vi "GCSTranslateError.vi"(5 "error in":errorcluster) -> (14 "GCS Error?":bool, 15 "Error Description":string, 19 "error out":errorcluster)   [LabVIEW 2009]
doc: "Returns if error in contains a GCS error code and if this is the \ncase, it displays the corresponding error message and \nappends it to \"source\" in \"error out\".\n\nValid for all systems"
panel:
  # "Returns if error in contains a GCS error code and if this is the \ncase, it displays the corresponding error message and \nappends it to \"source\" in \"error out\"."
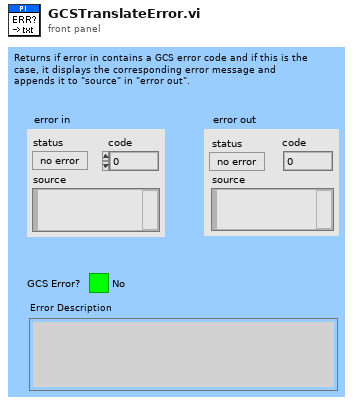
[diagram p1: front panel]
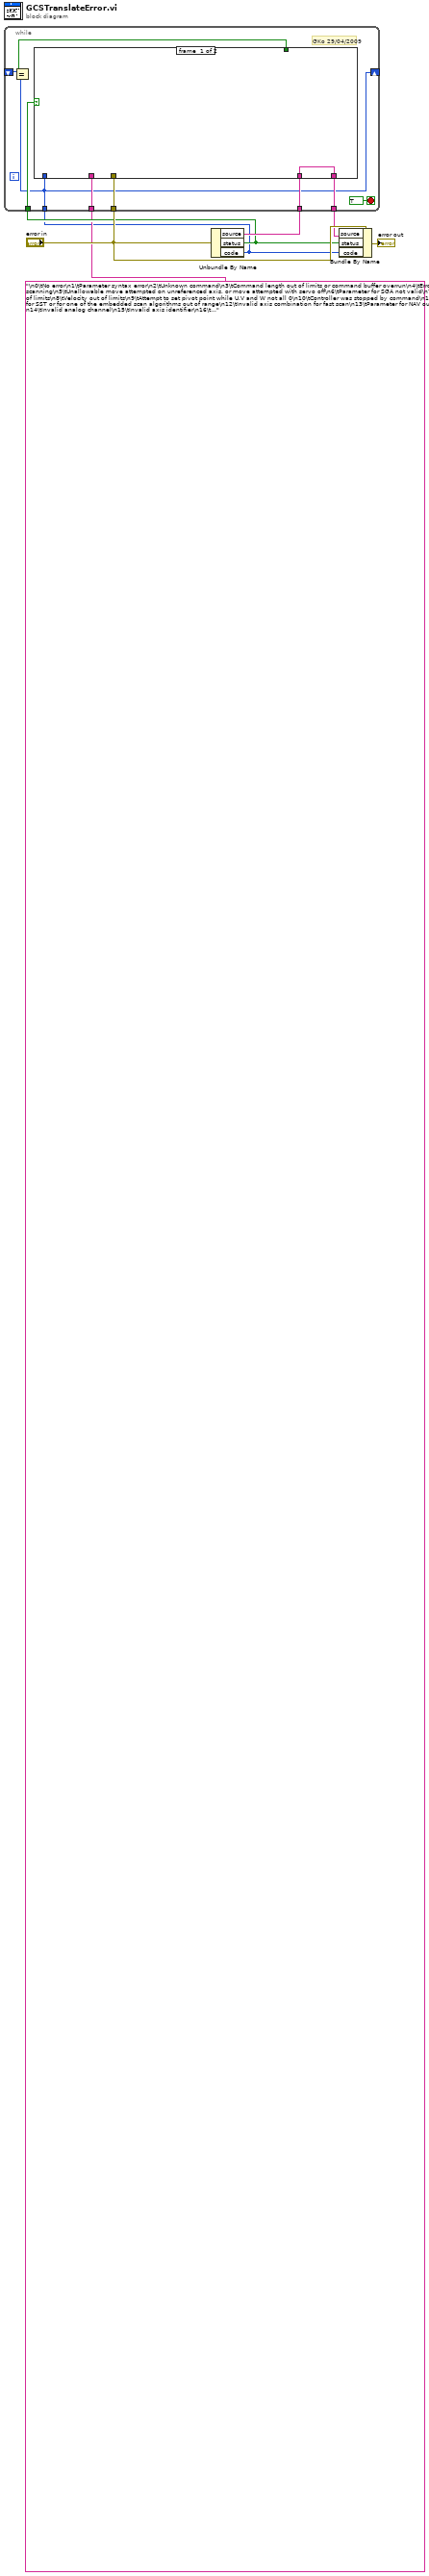
[diagram p0: block diagram]
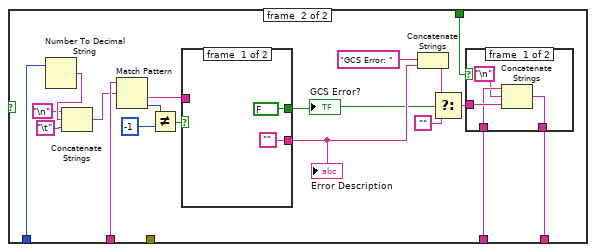
[diagram p2: hidden frame]
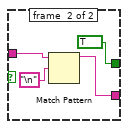
[diagram p4: hidden frame]
diagram:
  n1 = Unbundle By Name("error in") -> ("source"=w7:string, "status"=w3:bool, "code"=w1:i32)
  n2 = while {
    tunnel: w7 -> [w16]
    tunnel: "error in" -> [w15]
    tunnel: [w14] -> w4
    tunnel: w3 -> [w13]
    tunnel: w1 -> [w9]
    tunnel: "\n0\tNo error\n1\tParameter syntax error\n2\tUnknown command\n3\tCommand length out of limits or command buffer overrun\n4\tError while scanning\n5\tUnallowable move attempted on unreferenced axis, or move attempted with servo off\n6\tParameter for SGA not valid\n7\tPosition out of limits\n8\tVelocity out of limits\n9\tAttempt to set pivot point while U,V and W not all 0\n10\tController was stopped by command\n11\tParameter for SST or for one of the embedded scan algorithms out of range\n12\tInvalid axis combination for fast scan\n13\tParameter for NAV out of range\n14\tInvalid analog channel\n15\tInvalid axis identifier\n16\tUnknown stage name\n17\tParameter out of range\n18\tInvalid macro name\n19\tError while recording macro\n20\tMacro not found\n21\tAxis has no brake\n22\tAxis identifier specified more than once\n23\tIllegal axis\n24\tIncorrect number of parameters\n25\tInvalid floating point number\n26\tParameter missing\n27\tSoft limit out of range\n28\tNo manual pad found\n29\tNo more step-response values\n30\tNo step-response values recorded\n31\tAxis has no reference sensor\n32\tAxis has no limit switch\n33\tNo relay card installed\n34\tCommand not allowed for selected stage(s)\n35\tNo digital input installed\n36\tNo digital output configured\n37\tNo more MCM responses\n38\tNo MCM values recorded\n39\tController number invalid\n40\tNo joystick configured\n41\tInvalid axis for electronic gearing, axis can not be slave\n42\tPosition of slave axis is out of range\n43\tSlave axis cannot be commanded directly when electronic gearing is enabled\n44\tCalibration of joystick failed\n45\tReferencing failed\n46\tOPM (Optical Power Meter) missing\n47\tOPM (Optical Power Meter) not initialized or cannot be initialized\n48\tOPM (Optical Power Meter) Communication Error\n49\tMove to limit switch failed\n50\tAttempt to reference axis with referencing disabled\n51\tSelected axis is controlled by joystick\n52\tController detected communication error\n53\tMOV! motion still in progress\n54\tUnknown parameter\n55\tNo commands were recorded with REP\n56\tPassword invalid\n57\tData Record Table does not exist\n58\tSource does not exist; number too low or too high\n59\tSource Record Table number too low or too high\n60\tProtected Param: current Command Level (CCL) too low\n61\tCommand execution not possible while Autozero is running\n62\tAutozero requires at least one linear axis\n63\tInitialization still in progress\n64\tParameter is read-only\n65\tParameter not found in non-volatile memory\n66\tVoltage out of limits\n67\tNot enough memory available for requested wave curve\n68\tNot enough memory available for DDL table; DDL can not be started\n69\tTime delay larger than DDL table; DDL can not be started\n70\tThe requested arrays have different lengths; query them separately\n71\tAttempt to restart the generator while it is running in single step mode\n72\tMotion commands and wave generator activation are not allowed when analog target is active\n73\tMotion commands are not allowed when wave generator output is active; use WGO to disable generator output\n74\tNo sensor channel or no piezo channel connected to selected axis (sensor and piezo matrix)\n75\tGenerator started (WGO) without having selected a wave table (WSL).\n76\tInterface buffer did overrun and command couldn't be received correctly\n77\tData Record Table does not hold enough recorded data\n78\tData Record Table is not configured for recording\n79\tOpen-loop commands (SVA, SVR) are not allowed when servo is on\n80\tHardware error affecting RAM\n81\tNot macro command\n82\tMacro counter out of range\n83\tJoystick is active\n84\tMotor is off\n85\tMacro-only command\n86\tInvalid joystick axis\n87\tJoystick unknown\n88\tMove without referenced stage\n89\tCommand not allowed in current motion mode\n100\tPI LabVIEW driver reports error. See source control for details.\n200\tNo stage connected to axis\n201\tFile with axis parameters not found\n202\tInvalid axis parameter file\n203\tBackup file with axis parameters not found\n204\tPI internal error code 204\n205\tSMO with servo on\n206\tuudecode: incomplete header\n207\tuudecode: nothing to decode\n208\tuudecode: illegal UUE format\n209\tCRC32 error\n210\tIllegal file name (must be 8-0 format)\n211\tFile not found on controller\n212\tError writing file on controller\n213\tVEL command not allowed in DTR Command Mode\n214\tPosition calculations failed\n215\tThe connection between controller and stage may be broken\n216\tThe connected stage has driven into a limit switch, call CLR to resume operation\n217\tStrut test command failed because of an unexpected strut stop\n218\tWhile MOV! is running position can only be estimated!\n219\tPosition was calculated during MOV motion\n230\tInvalid handle\n231\tNo bios found\n232\tSave system configuration failed\n233\tLoad system configuration failed\n301\tSend buffer overflow\n302\tVoltage out of limits\n303\tOpen-loop motion attempted when servo ON\n304\tReceived command is too long\n305\tError while reading/writing EEPROM\n306\tError on I2C bus\n307\tTimeout while receiving command\n308\tA lengthy operation has not finished in the expected time\n309\tInsufficient space to store macro\n310\tConfiguration data has old version number\n311\tInvalid configuration data\n333\tInternal hardware error\n400\tWave generator index error\n401\tWave table not defined\n402\tWave type not supported\n403\tWave length exceeds limit\n404\tWave parameter number error\n405\tWave parameter out of range\n406\tWGO command bit not supported\n555\tBasMac: unknown controller error\n601\tNot enough memory\n602\tHardware voltage error\n603\tHardware temperature out of range\n1000\tToo many nested macros\n1001\tMacro already defined\n1002\tMacro recording not activated\n1003\tInvalid parameter for MAC\n1004\tDeleting macro failed\n1005\tController is busy with some lengthy operation (e.g. reference move, fast scan algorithm)\n2000\tController already has a serial number\n4000\tSector erase failed\n4001\tFlash program failed\n4002\tFlash read failed\n4003\tHW match code missing/invalid\n4004\tFW match code missing/invalid\n4005\tHW version missing/invalid\n4006\tFW version missing/invalid\n4007\tFW update failed\n0\tNo error occurred during function call\n-1\tError during com operation (could not be specified)\n-2\tError while sending data\n-3\tError while receiving data\n-4\tNot connected (no port with given ID open)\n-5\tBuffer overflow\n-6\tError while opening port\n-7\tTimeout error\n-8\tThere are more lines waiting in buffer\n-9\tThere is no interface or DLL handle with the given ID\n-10\tEvent/message for notification could not be opened\n-11\tFunction not supported by this interface type\n-12\tError while sending \"echoed\" data\n-13\tIEEE488: System error\n-14\tIEEE488: Function requires GPIB board to be CIC\n-15\tIEEE488: Write function detected no listeners\n-16\tIEEE488: Interface board not addressed correctly\n-17\tIEEE488: Invalid argument to function call\n-18\tIEEE488: Function requires GPIB board to be SAC\n-19\tIEEE488: I/O operation aborted\n-20\tIEEE488: Interface board not found\n-21\tIEEE488: Error performing DMA\n-22\tIEEE488: I/O operation started before previous operation completed\n-23\tIEEE488: No capability for intended operation\n-24\tIEEE488: File system operation error\n-25\tIEEE488: Command error during device call\n-26\tIEEE488: Serial poll-status byte lost\n-27\tIEEE488: SRQ remains asserted\n-28\tIEEE488: Return buffer full\n-29\tIEEE488: Address or board locked\n-30\tRS-232: 5 data bits with 2 stop bits is an invalid combination, as is 6, 7, or 8 data bits with 1.5 stop bits\n-31\tRS-232: Error configuring the COM port\n-32\tError dealing with internal system resources (events, threads, ...)\n-33\tA DLL or one of the required functions could not be loaded\n-34\tFTDIUSB: invalid handle\n-35\tFTDIUSB: device not found\n-36\tFTDIUSB: device not opened\n-37\tFTDIUSB: IO error\n-38\tFTDIUSB: insufficient resources\n-39\tFTDIUSB: invalid parameter\n-40\tFTDIUSB: invalid baud rate\n-41\tFTDIUSB: device not opened for erase\n-42\tFTDIUSB: device not opened for write\n-43\tFTDIUSB: failed to write device\n-44\tFTDIUSB: EEPROM read failed\n-45\tFTDIUSB: EEPROM write failed\n-46\tFTDIUSB: EEPROM erase failed\n-47\tFTDIUSB: EEPROM not present\n-48\tFTDIUSB: EEPROM not programmed\n-49\tFTDIUSB: invalid arguments\n-50\tFTDIUSB: not supported\n-51\tFTDIUSB: other error\n-52\tError while opening the COM port: was already open\n-53\tChecksum error in received data from COM port\n-54\tSocket not ready, you should call the function again\n-55\tPort is used by another socket\n-56\tSocket not connected (or not valid)\n-57\tConnection terminated (by peer)\n-58\tCan't connect to peer\n-59\tOperation was interrupted by a nonblocked signal\n-60\tNo Device with this ID is present\n-61\tDriver could not be opened (on Vista: run as administrator!)\n-1001\tUnknown axis identifier\n-1002\tNumber for NAV out of range--must be in [1,10000]\n-1003\tInvalid value for SGA--must be one of 1, 10, 100, 1000\n-1004\tController sent unexpected response\n-1005\tNo manual control pad installed, calls to SMA and related commands are not allowed\n-1006\tInvalid number for manual control pad knob\n-1007\tAxis not currently controlled by a manual control pad\n-1008\tController is busy with some lengthy operation (e.g. reference move, fast scan algorithm)\n-1009\tInternal error--could not start thread\n-1010\tController is (already) in macro mode--command not valid in macro mode\n-1011\tController not in macro mode--command not valid unless macro mode active\n-1012\tCould not open file to write or read macro\n-1013\tNo macro with given name on controller, or macro is empty\n-1014\tInternal error in macro editor\n-1015\tOne or more arguments given to function is invalid (empty string, index out of range, ...)\n-1016\tAxis identifier is already in use by a connected stage\n-1017\tInvalid axis identifier\n-1018\tCould not access array data in COM server\n-1019\tRange of array does not fit the number of parameters\n-1020\tInvalid parameter ID given to SPA or SPA?\n-1021\tNumber for AVG out of range--must be >0\n-1022\tIncorrect number of samples given to WAV\n-1023\tGeneration of wave failed\n-1024\tMotion error while axis in motion, call CLR to resume operation\n-1025\tController is (already) running a macro\n-1026\tConfiguration of PZT stage or amplifier failed\n-1027\tCurrent settings are not valid for desired configuration\n-1028\tUnknown channel identifier\n-1029\tError while reading/writing wave generator parameter file\n-1030\tCould not find description of wave form. Maybe WG.INI is missing?\n-1031\tThe WGWaveEditor DLL function was not found at startup\n-1032\tThe user cancelled a dialog\n-1033\tError from C-844 Controller\n-1034\tDLL necessary to call function not loaded, or function not found in DLL\n-1035\tThe open parameter file is protected and cannot be edited\n-1036\tThere is no parameter file open\n-1037\tSelected stage does not exist\n-1038\tThere is already a parameter file open. Close it before opening a new file\n-1039\tCould not open parameter file\n-1040\tThe version of the connected controller is invalid\n-1041\tParameter could not be set with SPA--parameter not defined for this controller!\n-1042\tThe maximum number of wave definitions has been exceeded\n-1043\tThe maximum number of wave generators has been exceeded\n-1044\tNo wave defined for specified axis\n-1045\tWave output to axis already stopped/started\n-1046\tNot all axes could be referenced\n-1047\tCould not find parameter set required by frequency relation\n-1048\tCommand ID given to SPP or SPP? is not valid\n-1049\tA stage name given to CST is not unique\n-1050\tA uuencoded file transfered did not start with \"begin\" followed by the proper filename\n-1051\tCould not create/read file on host PC\n-1052\tChecksum error when transfering a file to/from the controller\n-1053\tThe PiStages.dat database could not be found. This file is required to connect a stage with the CST command\n-1054\tNo wave being output to specified axis\n-1055\tInvalid password\n-1056\tError during communication with OPM (Optical Power Meter), maybe no OPM connected\n-1057\tWaveEditor: Error during wave creation, incorrect number of parameters\n-1058\tWaveEditor: Frequency out of range\n-1059\tWaveEditor: Error during wave creation, incorrect index for integer parameter\n-1060\tWaveEditor: Error during wave creation, incorrect index for floating point parameter\n-1061\tWaveEditor: Error during wave creation, could not calculate value\n-1062\tWaveEditor: Graph display component not installed\n-1063\tUser Profile Mode: Command is not allowed, check for required preparatory commands\n-1064\tUser Profile Mode: First target position in User Profile is too far from current position\n-1065\tController is (already) in User Profile Mode\n-1066\tUser Profile Mode: Block or Data Set index out of allowed range\n-1067\tProfileGenerator: No profile has been created yet\n-1068\tProfileGenerator: Generated profile exceeds limits of one or both axes\n-1069\tProfileGenerator: Unknown parameter ID in Set/Get Parameter command\n-1070\tProfileGenerator: Parameter out of allowed range\n-1071\tUser Profile Mode: Out of memory\n-1072\tUser Profile Mode: Cluster is not assigned to this axis\n-1073\tUnknown cluster identifier\n-1074\tThe installed device driver doesn't match the required version. Please see the documentation to determine the required device driver version.\n-1075\tThe library used doesn't match the required version. Please see the documentation to determine the required library version.\n-1076\tThe interface is currently locked by another function. Please try again later.\n" -> [w12]
    shift-right: [w9] -> _
    shift-left: _ -> [w10]
    stop <- TRUE stop-if-true
    # "GKo 29/04/2009"
    n3 = Equal?(x=w10, y=w9) -> (x = y?=w8:bool)
    n4 = case shown="True" w13 {
      tunnel: w16 -> [w17 w19]
      tunnel: w15 -> [_ _]
      tunnel: [w17 w35] -> w14
      tunnel: w12 -> [_ w31]
      tunnel: w9 -> [_ w24]
      tunnel: w8 -> [_ w18]
      frame #0 {
      }
      frame #1 {
        n5 = Number To Decimal String(number=w24) -> (decimal integer string=w30:string)  [unwired: 1 in]
        n6 = Concatenate Strings("\n" ("string"), w30, "\t" ("string")) -> (w27:string)
        n7 = Match Pattern(string=w31, regular expression=w27) -> (after substring=w26:string, offset past match=w23:i32)  [unwired: 1 in, 2 out]
        n8 = Not Equal?(x=w23, y=-1) -> (x != y?=w21:bool)
        n9 = case shown="False" w21 {
          tunnel: w26 -> [_ w47]
          tunnel: ["" w45] -> w25
          tunnel: [FALSE TRUE] -> w20
          frame #0 {
          }
          frame #1 {
            n10 = Match Pattern(string=w47, regular expression="\n" ("string")) -> (before substring=w45:string)  [unwired: 1 in, 3 out]
          }
        }
        "Error Description" <- w25
        "GCS Error?" <- w20
        n11 = Concatenate Strings("GCS Error: " ("Substring"), w25) -> (w33:string)
        n12 = Select(t=w33, s=w20, f="") -> (s? t:f=w32:string)
        n13 = case shown="False" w18 {
          tunnel: [w40 w41] -> w35
          tunnel: w32 -> [w39 _]
          tunnel: w19 -> [w38 w41]
          frame #0 {
            n14 = Concatenate Strings(w38, "\n", w39) -> (w40:string)
          }
          frame #1 {
          }
        }
      }
    }
  }
  n15 = Bundle By Name(cluster="error in", "source"=w4, "status"=w3, "code"=w1) -> (→"error out":errorcluster)
